vi "Front-load.vi"(5 "Show UI?(F)":bool, 7 "Load Interrupt":refnum<notifier>, 8 "error in (no error)":errorcluster, 11 "Scope(Paths)":T1) -> (0 "error out":errorcluster, 1 "Success?":bool)   [LabVIEW 2019, in "ClassLoader.lvlib"]
doc: "Front-load data. This will scan for new PPLs (using 'Register PPLs.vi') as well as load the cached data.\nCan be interrupted using the 'Load Interrupt'. Can show a UI.\n\nThe Scope determined how much of the cached data will be loaded."
uses:
  ClassLoader.lvlib
  Sub/Ctl/Ctl_Front-load Scope.ctl
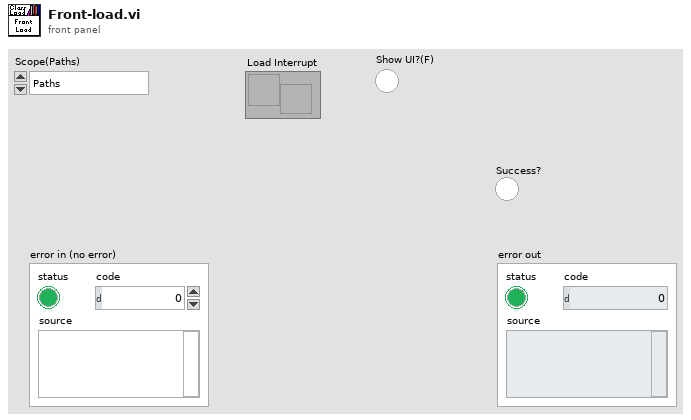
[diagram p1: front panel]
types:
  T1 = typedef "ClassLoader.lvlib/Ctl_Front-load Scope.ctl" = enum16{"Paths", "Paths and Hierarchies", "All"}
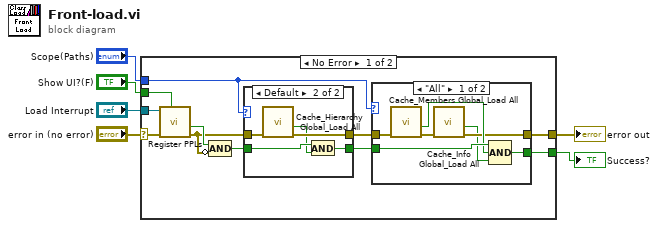
[diagram p0: block diagram]
diagram:
  n1 = case shown="No Error" "error in (no error)" {
    selector: "error in (no error)" -> [w17 w34]
    tunnel: [w11 w34] -> w5
    tunnel: [w9 _] -> w4
    tunnel: "Show UI?(F)" -> [w15 _]
    tunnel: "Load Interrupt" -> [w14 _]
    tunnel: "Scope(Paths)" -> [w10 _]
    frame No Error {
      n2 = call "Register PPLs.vi"("Show UI?(F)"=w15, "error in"=w17, "Interrupt"=w14) -> ("error out"=w13:errorcluster, "Success?"=w16:bool)  [unwired: 7 in]
      n3 = Compound Arithmetic op=AND(w16, invert w13) -> (w8:bool)
      n4 = case shown="Default" w10 {
        tunnel: [w28 w33] -> w12
        tunnel: w13 -> [w28 w32]
        tunnel: w8 -> [w27 w31]
        tunnel: [w27 w29] -> w7
        frame "Paths" {
        }
        frame Default {
          n5 = call "Cache_Hierarchy Global_Load All.vi"("error in (no error)"=w32) -> ("error out"=w33:errorcluster, "All Success?"=w30:bool)  [unwired: 8 in, 1 out]
          n6 = And(x=w31, y=w30) -> (x .and. y?=w29:bool)
        }
      }
      n7 = case shown="\"All\"" w10 {
        tunnel: [w19 w26] -> w11
        tunnel: w12 -> [w24 w26]
        tunnel: [w21 w25] -> w9
        tunnel: w7 -> [w23 w25]
        frame "All" {
          n8 = call "Cache_Members Global_Load All.vi"("error in (no error)"=w24) -> ("error out"=w20:errorcluster, "All Success?"=w22:bool)  [unwired: 8 in, 1 out]
          n9 = call "Cache_Info Global_Load All.vi"("error in (no error)"=w20) -> ("error out"=w19:errorcluster, "All Success?"=w18:bool)  [unwired: 7 in, 2 out]
          n10 = Compound Arithmetic op=AND(w23, w22, w18) -> (w21:bool)
        }
        frame Default {
        }
      }
    }
    frame Error {
    }
  }
  "error out" <- w5
  "Success?" <- w4
